vi "throw from error.vi"(5 "call chain?":bool, 6 "context":T1, 7 "source":string, 8 "error in":errorcluster, 9 "message":string, 10 "severity":T2, 11 "code":i32) -> (0 "exception out":T3 {"code" format="%.0x"})   [LabVIEW 2013, in "exception.lvlib"]
uses:
  exception.lvlib
  exception.ctl
  context.ctl
  severity.ctl
  const sourcename.vi
  const severityname.vi
  const messagename.vi
  const exceptioncausename.vi
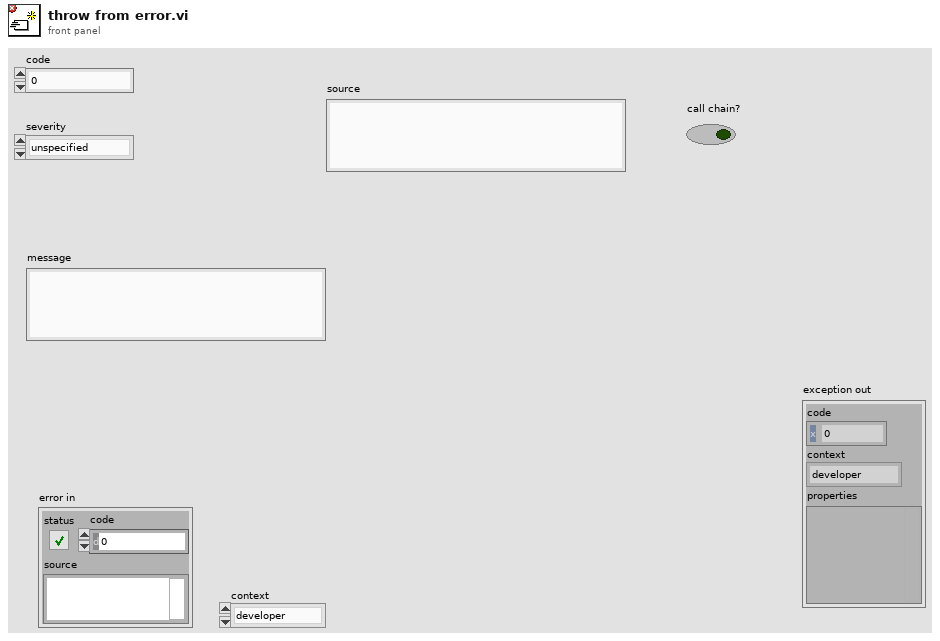
[diagram p1: front panel]
types:
  T1 = typedef "exception.lvlib/context.ctl" = enum16{"developer", "user interface", "standard", "limited", "deterministic"}
  T2 = typedef "exception.lvlib/severity.ctl" = enum8{"unspecified", "informational", "operation failed", "data corruption", "system corruption", "critical unknown state"}
  T3 = typedef "exception.lvlib/exception.ctl" = cluster{"code":i32, "context":T1, "properties":variant}
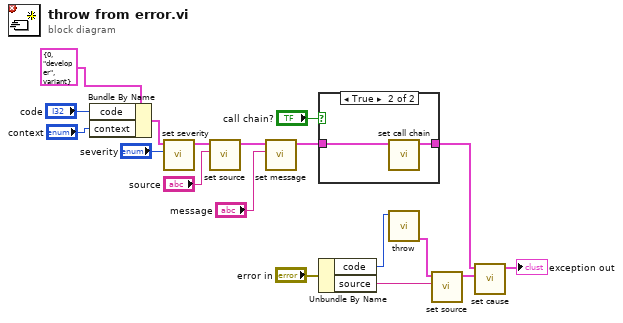
[diagram p0: block diagram]
diagram:
  n1 = Bundle By Name(cluster=T3 {"code"=0, "context"=enum."developer", "properties"=variant} ("exception"), "code"="code", "context"="context") -> (w17:T3)
  n2 = call "set severity.vi"("severity"="severity", "exception in"=w17) -> ("exception out"=w9:T3)  [unwired: 9 in]
  n3 = call "set source.vi"("source"="source", "exception in"=w9) -> ("exception out"=w15:T3)  [unwired: 9 in]
  n4 = call "set message.vi"("message"="message", "exception in"=w15) -> ("exception out"=w13:T3)  [unwired: 9 in]
  n5 = case shown="True" "call chain?" {
    tunnel: w13 -> [w19 w21]
    tunnel: [w19 w20] -> w10
    frame False {
    }
    frame True {
      n6 = call "set call chain.vi"("exception in"=w21) -> ("exception out"=w20:T3)  [unwired: 10 in]
    }
  }
  n7 = Unbundle By Name("error in") -> ("code"=w5:i32, "source"=w6:string)
  n8 = call "throw.vi"("code"=w5) -> ("exception"=w4:T3)  [unwired: 10 in]
  n9 = call "set source.vi"("source"=w6, "exception in"=w4) -> ("exception out"=w1:T3)  [unwired: 9 in]
  n10 = call "set cause.vi"("cause"=w1, "exception in"=w10) -> ("exception out"=→"exception out":T3)  [unwired: 9 in]
